vi "create_all_data_queue.vi"(8 "error in (no error)":errorcluster) -> (0 "error out":errorcluster, 3 "data_queues":T1)   [LabVIEW 2017]
uses:
  all_data_queue.ctl
  measurement_data/MeasurementDatalvclass.lvclass
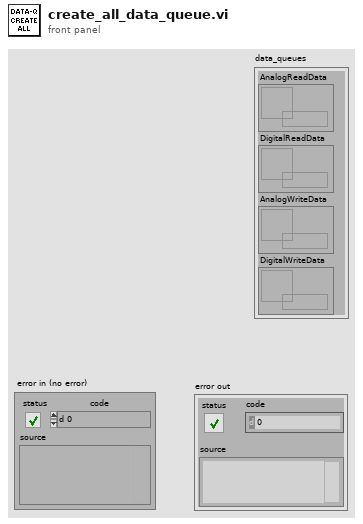
[diagram p1: front panel]
types:
  T1 = typedef "all_data_queue.ctl" = cluster{"AnalogReadData":refnum<queue>, "DigitalReadData":refnum<queue>, "AnalogWriteData":refnum<queue>, "DigitalWriteData":refnum<queue>}
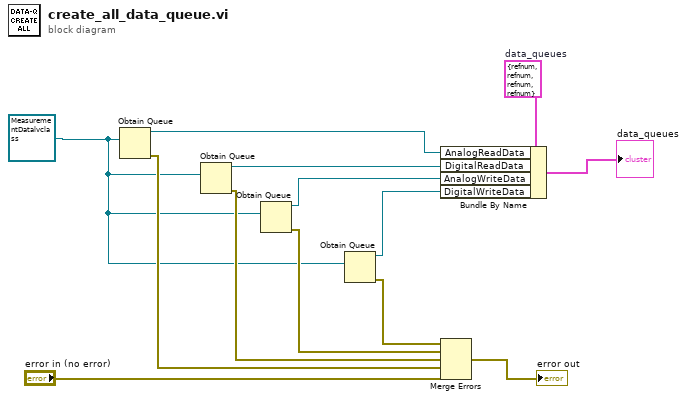
[diagram p0: block diagram]
diagram:
  w1 = refnum<class "MeasurementDatalvclass.lvclass"> refnum ("MeasurementDatalvclass.lvclass")
  w10 = T1 {"AnalogReadData"=refnum, "DigitalReadData"=refnum, "AnalogWriteData"=refnum, "DigitalWriteData"=refnum}  # data_queues
  n1 = Obtain Queue(element data type=w1) -> (queue out=w13:refnum<queue>, error out=w8:errorcluster)  [unwired: 4 in, 1 out]
  n2 = Obtain Queue(element data type=w1) -> (queue out=w7:refnum<queue>, error out=w6:errorcluster)  [unwired: 4 in, 1 out]
  n3 = Obtain Queue(element data type=w1) -> (queue out=w5:refnum<queue>, error out=w3:errorcluster)  [unwired: 4 in, 1 out]
  n4 = Obtain Queue(element data type=w1) -> (queue out=w4:refnum<queue>, error out=w2:errorcluster)  [unwired: 4 in, 1 out]
  n5 = Bundle By Name(cluster=w10, "AnalogReadData"=w13, "DigitalReadData"=w7, "AnalogWriteData"=w5, "DigitalWriteData"=w4) -> (→"data_queues":T1)
  n6 = Merge Errors(w2, w3, w6, w8, "error in (no error)") -> (→"error out":errorcluster)
